vi "Pre Launch Init.vi"(11 "uService Template in":refnum<class "Common GUI v3.lvclass">) -> (0 "error out":errorcluster, 3 "uService Template out":refnum<class "Common GUI v3.lvclass">)   [LabVIEW 2026, in "TALOS.lvlib" / "Common GUI v3.lvlib" / "Common GUI v3.lvclass"]
doc: "(<B>Filename</B>: Actor Framework.lvlib:Actor.lvclass:Pre Launch Init.vi)\n\nDefines behavior that occurs after the Launch Nested Actor method is invoked but before the actor's Actor Core method begins running.\n\nBy default, this method does nothing. A descendant class may override it to define behavior."
uses:
  Common GUI v3.lvclass
  Common GUI v3.lvclass/Common GUI v3.ctl
  Father of all uServices/Father of all uServices/Father of all uServices.lvclass
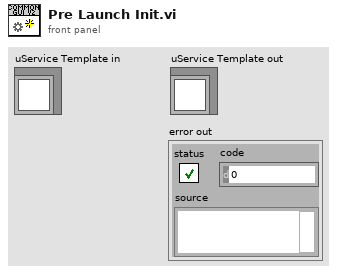
[diagram p1: front panel]
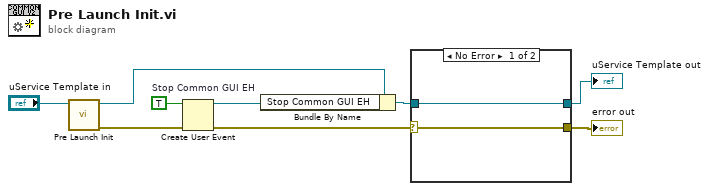
[diagram p0: block diagram]
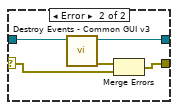
[diagram p2: hidden frame]
diagram:
  w8 = TRUE  # Stop Common GUI EH
  n1 = call-parent "Pre Launch Init.vi"("uService Template in"="uService Template in") -> ("error out"=w5:errorcluster, "uService Template out"=w7:refnum<class "Common GUI v3.lvclass">)  [unwired: 9 in]
  n2 = Create User Event(user event datatype=w8, error in=w5) -> (user event=w6:refnum<user-event>, error out=w4:errorcluster)
  n3 = Bundle By Name(cluster=w7, "Stop Common GUI EH"=w6) -> (w3:refnum<class "Common GUI v3.lvclass">)
  n4 = case shown="No Error" w4 {
    selector: w4 -> [w11 w12]
    tunnel: w3 -> [w10 w16]
    tunnel: [w11 w13] -> w1
    tunnel: [w10 w14] -> w2
    frame No Error {
    }
    frame Error {
      n5 = call "Destroy Events - Common GUI v3.vi"("Common GUI uService in"=w16) -> ("error out"=w15:errorcluster, "Common GUI uService out"=w14:refnum<class "Common GUI v3.lvclass">)  [unwired: 9 in]
      n6 = Merge Errors(w15, w12) -> (w13:errorcluster)
    }
  }
  "error out" <- w1
  "uService Template out" <- w2
